vi "transmitPicture.vi"(8 "error in (no error)":errorcluster, 11 "24-bit pixmap":u32[][](array[numeric])) -> (0 "error out":errorcluster)   [LabVIEW 2014]
uses:
  typeDefs/pixxelAction.ctl
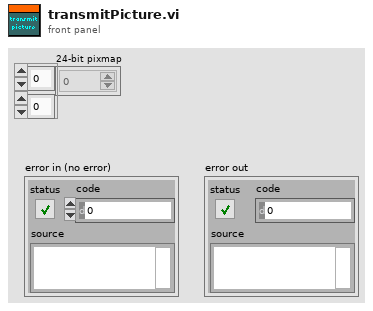
[diagram p1: front panel]
types:
  T1 = typedef "pixxelAction.ctl" = enum16{"init", "watchdog", "headScene", "setPixel", "tailScene", "headProg", "tailProg", "showSceneFrame", "black", "playFrames", "close", "uploadProg", "startProg", "pauseProg", "stopProg", "jumpTo", "setIP", "setGW", "initFlash", "saveScene", "saveProgram"}
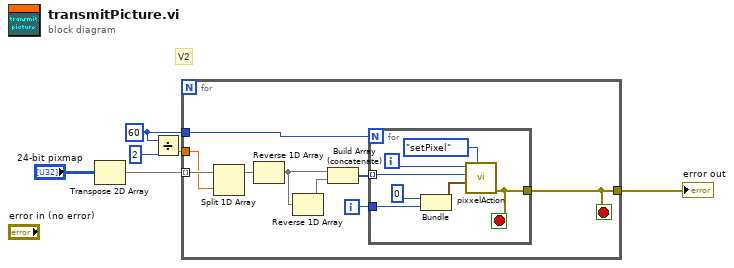
[diagram p0: block diagram]
diagram:
  w2 = 60
  # "V2"
  n1 = Transpose 2D Array(2D array="24-bit pixmap") -> (transposed array=w6:u32[][])
  n2 = Divide(x=w2, y=2) -> (x/y=w4:dbl)
  n3 = for {
    tunnel: w6 -> [w13] mode=indexing
    tunnel: [w7] -> w5
    tunnel: w2 -> [w14]
    tunnel: w4 -> [w9]
    i -> [w15]
    stop <- w7 stop-if-true
    n4 = Split 1D Array(array=w13, index=w9) -> (first subarray=w11:u32[])  [unwired: 1 out]
    n5 = Reverse 1D Array(array=w11) -> (reversed array=w8:u32[])
    n6 = Reverse 1D Array(array=w8) -> (reversed array=w12:u32[])
    n7 = Build Array (concatenate)(w8, w12) -> (w10:u32[])
    n8 = for {
      N: w14 -> [_]
      tunnel: w10 -> [w22] mode=indexing
      tunnel: w15 -> [w17]
      tunnel: [w16] -> w7
      i -> [w18]
      stop <- w16 stop-if-true
      n9 = Bundle(0, w17) -> (w20:cluster{i32, i32})  [unwired: 1 in]
      n10 = call "pixxelAction.vi"("PIXXELaction"=pixxelAction."setPixel", "location"=w20, "color"=w22, "Pixel-nummer"=w18) -> ("error out"=w16:errorcluster)  [unwired: 7 in]
    }
  }
  "error out" <- w5
